vi "Receive Boolean.vi"(8 "error in (no error)":errorcluster, 10 "Broadcast Boolean Msg":refnum<class "Broadcast Boolean Msg.lvclass">, 11 "ButtonPanel In":refnum<class "AutoRegPanel.lvclass">) -> (0 "error out":errorcluster, 3 "ButtonPanel Out":refnum<class "AutoRegPanel.lvclass">)   [LabVIEW 2015, in "TestActors.lvlib" / "AutoRegPanel.lvclass"]
uses:
  AutoRegPanel.lvclass
  IViewable/IViewable Messages/Broadcast Boolean Msg/Broadcast Boolean Msg.lvclass
  IViewable/IViewable Messages/Broadcast Boolean Msg/Broadcast Boolean Msg.lvclass/Broadcast Boolean Msg.ctl
  IViewable/IViewable/IViewable.lvclass
  Dialog Box Implementations/OneButtonDialogBox/OneButtonDialogBox.lvclass
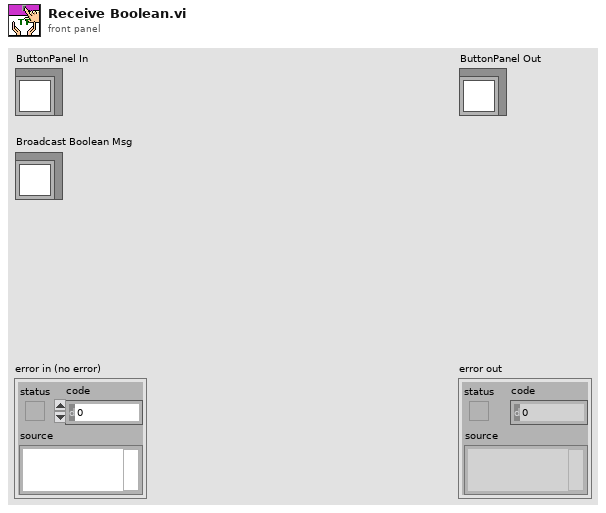
[diagram p1: front panel]
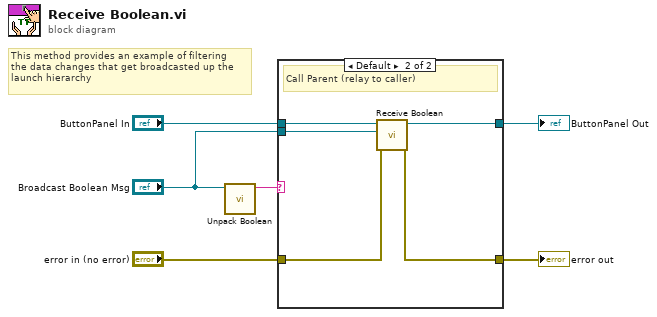
[diagram p0: block diagram]
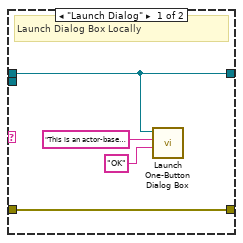
[diagram p2: hidden frame]
diagram:
  # "This method provides an example of filtering\nthe data changes that get broadcasted up the\nlaunch hierarchy"
  n1 = call "Unpack Boolean.vi"("Broadcast Boolean Msg In"="Broadcast Boolean Msg") -> ("Control Label"=w1:string)  [unwired: 9 in, 1 out]
  n2 = case shown="Default" w1 {
    tunnel: [w10 w15] -> w6
    tunnel: [w7 w14] -> w5
    tunnel: "error in (no error)" -> [w10 w13]
    tunnel: "ButtonPanel In" -> [w7 w12]
    tunnel: "Broadcast Boolean Msg" -> [_ w11]
    frame "Launch Dialog" {
      # "Launch Dialog Box Locally"
      n3 = call "Launch One-Button Dialog Box.vi"("Button Text (OK)"="OK" ("Button Text"), "Message Text"="This is an actor-based dialog box", "Dialog Launcher"=w7) -> ()  [unwired: 8 in, 1 out]
    }
    frame Default {
      # "Call Parent (relay to caller)"
      n4 = call-parent "Receive Boolean.vi"("error in (no error)"=w13, "Broadcast Boolean Msg"=w11, "IViewable In"=w12) -> ("error out"=w15:errorcluster, "IViewable Out"=w14:refnum<class "AutoRegPanel.lvclass">)  [unwired: 7 in]
    }
  }
  "error out" <- w6
  "ButtonPanel Out" <- w5
